vi "get_component_type_name.vi"(8 "error in (no error)":errorcluster, 11 "GenericDigitalOut in":refnum<class "GenericDigitalOut.lvclass">) -> (0 "error out":errorcluster, 2 "String":string, 3 "GenericDigitalOut out":refnum<class "GenericDigitalOut.lvclass">)   [LabVIEW 2010, in "GenericDigitalOut.lvclass"]
uses:
  GenericDigitalOut.lvclass
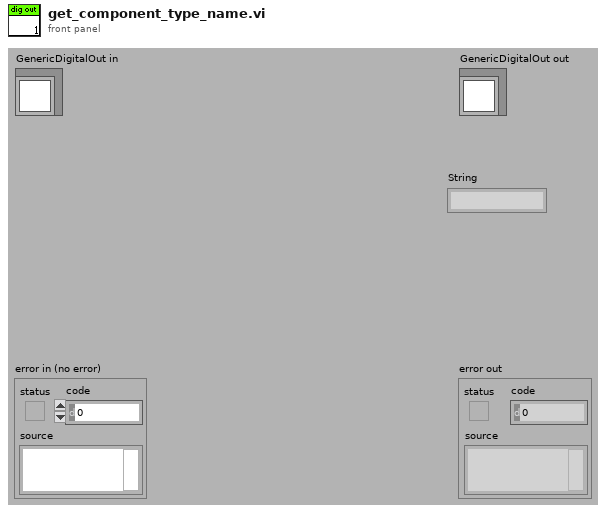
[diagram p1: front panel]
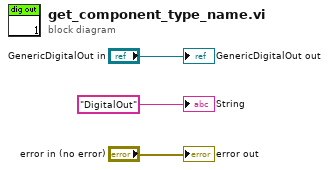
[diagram p0: block diagram]
diagram:
  "error out" <- "error in (no error)"
  "GenericDigitalOut out" <- "GenericDigitalOut in"
  "String" <- "DigitalOut" ("String")
